vi "remote.Execute Generic Command.vi"(0 "SLSC Remote in":refnum<class "SLSC Interface.lvclass">, 5 "resources":string, 7 "command":refnum<k21>, 11 "error in (no error)":errorcluster, 12 "timeout (10 sec)":dbl=10.0) -> (4 "SLSC Remote out":refnum<class "SLSC Interface.lvclass">, 15 "error out":errorcluster)   [LabVIEW 2016, in "SLSC Interface.lvclass"]
uses:
  SLSC Interface Class/SLSC Interface.lvclass
  SLSC Interface Class/SLSC Interface.lvclass/SLSC Interface.ctl
  SLSC Interface Class/Read client handle.vi
  SLSC Interface Class/Read URL.vi
  <vilib>/NI/JSON Support for LabVIEW/JSON Data Classes/JSON Object/JSON Object.lvclass
  C:/Program Files (x86)/National Instruments/LabVIEW 2016/vi.lib/NI/JSON Support for LabVIEW/JSON Data Classes/JSON Datatype/JSON Null.lvclass
  SLSC Interface Class/Read session.vi
  <vilib>/NI/JSON Support for LabVIEW/JSON Data Classes/JSON Object/New JSON Object (Empty).vi
  <vilib>/NI/JSON Support for LabVIEW/JSON Data Classes/JSON Object/Insert Key Value Pair (Single String).vi
  <vilib>/NI/JSON Support for LabVIEW/JSON Data Classes/JSON Object/Insert Key Value Pair (Single Numeric).vi
  <vilib>/NI/NI JSONRPC Server Framework/Classes/Server/Format Client Request (Auto-Increment).vi
  <vilib>/httpClient/POSTBuffer.vi
  <vilib>/NI/NI JSONRPC Server Framework/Classes/Server/Parse Response (Object).vi
  <vilib>/NI/NI JSONRPC Server Framework/Classes/Server/JSONRPC Server.lvclass
  <vilib>/httpClient/LabVIEWHTTPClient.lvlib
  <vilib>/NI/JSON Support for LabVIEW/JSON Data Classes/JSON Helper/JSON Helper.lvclass
  C:/Program Files (x86)/National Instruments/LabVIEW 2016/vi.lib/NI/JSON Support for LabVIEW/JSON Data Classes/JSON Structured Type/JSON Structure.lvclass
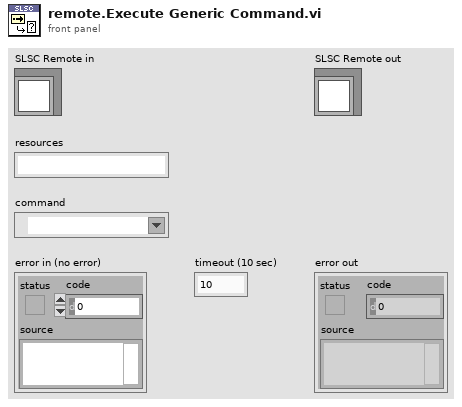
[diagram p1: front panel]
types:
  T1 = typedef "LabVIEWHTTPClient.lvlib/ClientHandle.ctl" = refnum<k1>
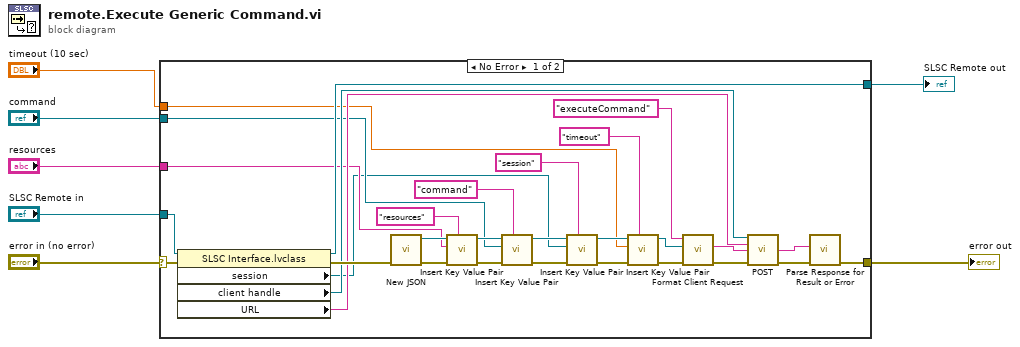
[diagram p0: block diagram]
diagram:
  n1 = case shown="No Error" "error in (no error)" {
    selector: "error in (no error)" -> [w35 w38]
    tunnel: "resources" -> [w15 _]
    tunnel: "SLSC Remote in" -> [w37 w39]
    tunnel: [w36 w39] -> w4
    tunnel: [w25 w38] -> w2
    tunnel: "command" -> [w14 _]
    tunnel: "timeout (10 sec)" -> [w12 _]
    frame No Error {
      n2 = property class="SLSC Interface.lvclass"(reference=w37, error in=w35) -> (reference out=w36:refnum<class "SLSC Interface.lvclass">, error out=w34:errorcluster, "session"=w13:refnum<k21>, "client handle"=w30:T1, "URL"=w29:string)
      n3 = call-poly <vilib>:"New JSON.vi"("error in (no error)"=w34) -> ("error out"=w33:errorcluster, "JSON Object out"=w19:refnum<class "JSON Object.lvclass">)  [unwired: 9 in]
      n4 = call-poly <vilib>:"Insert Key Value Pair.vi"("key"="resources" ("Name"), "error in (no error)"=w33, "value"=w15, "JSON Object in"=w19) -> ("error out"=w24:errorcluster, "JSON Object out"=w18:refnum<class "JSON Object.lvclass">)  [unwired: 5 in, 1 out]
      n5 = call-poly <vilib>:"Insert Key Value Pair.vi"("key"="command" ("Name"), "error in (no error)"=w24, "value"=w14, "JSON Object in"=w18) -> ("error out"=w23:errorcluster, "JSON Object out"=w17:refnum<class "JSON Object.lvclass">)  [unwired: 5 in, 1 out]
      n6 = call-poly <vilib>:"Insert Key Value Pair.vi"("key"="session" ("Name"), "error in (no error)"=w23, "value"=w13, "JSON Object in"=w17) -> ("error out"=w22:errorcluster, "JSON Object out"=w16:refnum<class "JSON Object.lvclass">)  [unwired: 5 in, 1 out]
      n7 = call-poly <vilib>:"Insert Key Value Pair.vi"("key"="timeout" ("Name"), "error in (no error)"=w22, "value"=w12, "JSON Object in"=w16) -> ("error out"=w20:errorcluster, "JSON Object out"=w21:refnum<class "JSON Object.lvclass">)  [unwired: 5 in, 1 out]
      n8 = call-poly <vilib>:"Format Client Request.vi"("error in (no error)"=w20, "JSON in"=w21, "method"="executeCommand") -> ("error out"=w28:errorcluster, "Request String"=w31:string)  [unwired: 7 in]
      n9 = call-poly <vilib>:"POST.vi"("client handle"=w30, "url"=w29, "buffer"=w31, "error in (no error)"=w28) -> ("body"=w27:string, "error out"=w26:errorcluster)  [unwired: 8 in, 2 out]
      n10 = call-poly <vilib>:"Parse Response for Result or Error.vi"("error in"=w26, "Response String In"=w27) -> ("error out"=w25:errorcluster)  [unwired: 7 in, 2 out]
    }
    frame Error {
    }
  }
  "error out" <- w2
  "SLSC Remote out" <- w4
